vi "Save Test Executive.vi"(8 "error in (no error)":errorcluster, 10 "Path":path, 11 "Test Executive Builder Model in":refnum<class "Test Executive Builder Model.lvclass">) -> (0 "error out":errorcluster, 3 "Test Executive Builder Model out":refnum<class "Test Executive Builder Model.lvclass">)   [LabVIEW 2017, in "Test Executive Builder Model.lvclass"]
uses:
  Test Executive Builder Model.lvclass
  <vilib>/gpm_packages/@cs/test-executive/Source/Test Executive/TestExecutive Ref/TestExecutive Ref.lvclass
  <vilib>/gpm_packages/@cs/mva-core/Source/IModel/IModel/IModel.lvclass
  C:/Users/jonmc/Documents/Git/Test Executive Builder/gpm_packages/@cs/mva-core/Source/IModel/IModel/IModel.lvclass
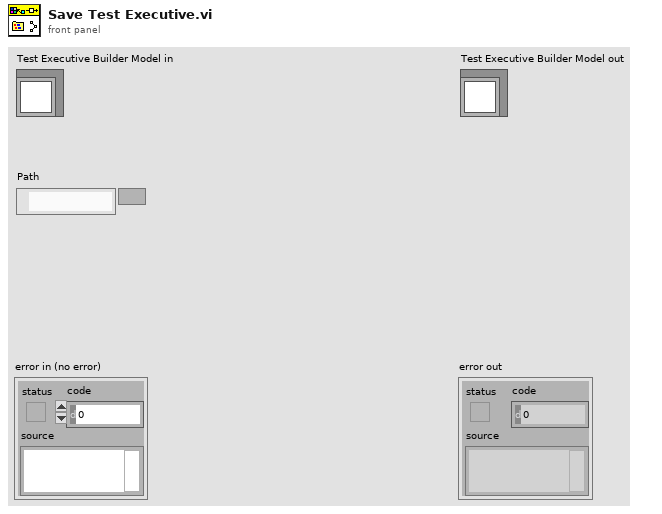
[diagram p1: front panel]
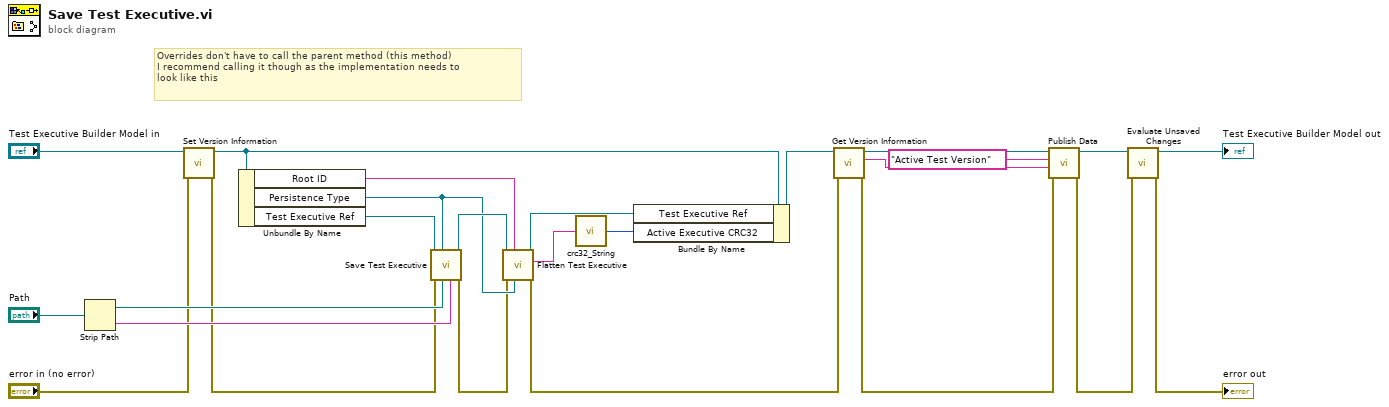
[diagram p0: block diagram]
diagram:
  # "Overrides don't have to call the parent method (this method)\nI recommend calling it though as the implementation needs to\nlook like this"
  n1 = Strip Path(path="Path") -> (stripped path=w23:path, name=w22:string)
  n2 = call-dynamic "Set Version Information.vi"("error in (no error)"="error in (no error)", "Test Executive Builder Model in"="Test Executive Builder Model in") -> ("error out"=w9:errorcluster, "Test Executive Builder Model out"=w10:refnum<class "Test Executive Builder Model.lvclass">)  [unwired: 8 in]
  n3 = Unbundle By Name(w10) -> ("Root ID"=w18:string, "Persistence Type"=w17:refnum<class "IPersist.lvclass">, "Test Executive Ref"=w24:refnum<data-value>)
  n4 = call <vilib>:"Save Test Executive.vi"("File Name"=w22, "Folder"=w23, "Persistence in"=w17, "error in (no error)"=w9, "Test Executive Ref"=w24) -> ("error out"=w16:errorcluster, "Test Executive Ref out"=w20:refnum<data-value>)  [unwired: 5 in]
  n5 = call <vilib>:"Flatten Test Executive.vi"("Persistence in"=w17, "Root ID"=w18, "error in (no error)"=w16, "Test Executive Ref"=w20) -> ("error out"=w3:errorcluster, "Flattened Test Executive"=w21:string, "Test Executive Ref out"=w19:refnum<data-value>)  [unwired: 5 in]
  n6 = call "crc32_String.vi"("String in"=w21) -> ("CRC32"=w15:u32)  [unwired: 1 in]
  n7 = Bundle By Name(cluster=w10, "Test Executive Ref"=w19, "Active Executive CRC32"=w15) -> (w5:refnum<class "Test Executive Builder Model.lvclass">)
  n8 = call-dynamic "Get Version Information.vi"("error in (no error)"=w3, "Test Executive Builder Model in"=w5) -> ("error out"=w2:errorcluster, "Version Info"=w6:string, "Test Executive Builder Model out"=w7:refnum<class "Test Executive Builder Model.lvclass">)  [unwired: 7 in]
  n9 = call <vilib>:"Publish Data.vi"("error in (no error)"=w2, "Data to Publish"=w6, "Datum Name"="Active Test Version", "IModel in"=w7) -> ("error out"=w1:errorcluster, "IModel out"=w4:refnum<class "Test Executive Builder Model.lvclass">)  [unwired: 6 in]
  n10 = call-dynamic "Evaluate Unsaved Changes.vi"("error in (no error)"=w1, "Test Executive Builder Model in"=w4) -> ("error out"=→"error out":errorcluster, "Test Executive Builder Model out"=→"Test Executive Builder Model out":refnum<class "Test Executive Builder Model.lvclass">)  [unwired: 8 in]
